vi "n!.vi"() -> ()   [LabVIEW 2015]
panel:
  out "n！":dbl format="%#_6f"
  out "n！":dbl
  in  "请输入":dbl
  # "For Loop范例"
  # "Feedback Node范例"
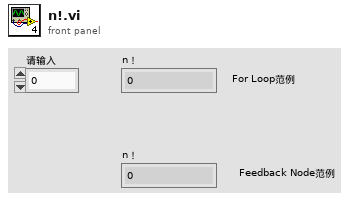
[diagram p1: front panel]
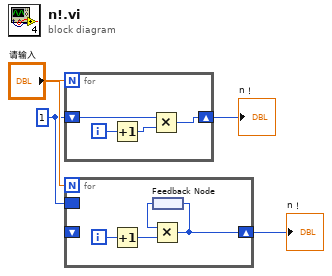
[diagram p0: block diagram]
diagram:
  w2 = 1
  n1 = for {
    N: "请输入" -> [_]
    shift-right: [w8] -> w4
    shift-left: w2 -> [w7]
    i -> [w6]
    n2 = Increment(x=w6) -> (x+1=w5:i32)
    n3 = Multiply(x=w7, y=w5) -> (x*y=w8:i32)
  }
  "n！" <- w4
  n4 = for {
    N: "请输入" -> [_]
    shift-right: [w10] -> w1
    shift-left: _ -> [_]
    border: w2 -> [_]
    i -> [w12]
    n5 = Increment(x=w12) -> (x+1=w11:i32)
    n6 = feedback #1() -> (w9:i32)
    n7 = Multiply(x=w9, y=w11) -> (x*y=w10:i32)
    n8 = feedback-in #1(w10) -> ()
  }
  "n！" <- w1
